vi "EnableDisable RTM.vi"(11 "Node Ptr":T1 format="%.0x") -> ()   [LabVIEW 2020, in "Ballard ARINC 429 System Explorer.lvlib" / "Implementation.lvlib"]
uses:
  Implementation.lvlib
  <vilib>/NI VeriStand/Custom Device API/Custom Device Item Ref.ctl
  Scripting/Ballard/Constants.vi
  <vilib>/NI VeriStand/Custom Device API/Custom Device API.lvlib
  Scripting/Ballard/Ballard ARINC 429 Scripting.lvlib
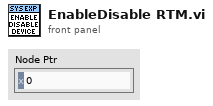
[diagram p1: front panel]
types:
  T1 = typedef "Custom Device API.lvlib/Custom Device Item Ref.ctl" = u64
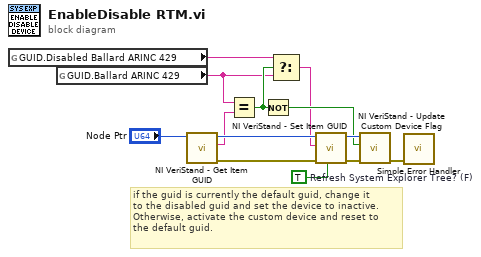
[diagram p0: block diagram]
diagram:
  w1 = TRUE  # Refresh System Explorer Tree? (F)
  # "if the guid is currently the default guid, change it \nto the disabled guid and set the device to inactive. \nOtherwise, activate the custom device and reset to \nthe default guid."
  n1 = global read "Constants.vi" "GUID.Disabled Ballard ARINC 429"() -> (w4:string)
  n2 = global read "Constants.vi" "GUID.Ballard ARINC 429"() -> (w3:string)
  n3 = call <vilib>:"NI VeriStand - Get Item GUID.vi"("Item Ref in"="Node Ptr") -> ("error out"=w9:errorcluster, "GUID"=w7:string, "Item Ref out"=w10:T1)  [unwired: 8 in]
  n4 = Equal?(x=w3, y=w7) -> (x = y?=w6:bool)
  n5 = Not(x=w6) -> (.not. x?=w5:bool)
  n6 = Select(t=w4, s=w6, f=w3) -> (s? t:f=w2:string)
  n7 = call <vilib>:"NI VeriStand - Set Item GUID.vi"("Refresh System Explorer Tree? (F)"=w1, "error in (no error)"=w9, "GUID"=w2, "Item Ref in"=w10) -> ("error out"=w8:errorcluster, "Item Ref out"=w11:T1)  [unwired: 6 in]
  n8 = call <vilib>:"NI VeriStand - Update Custom Device Flag.vi"("error in (no error)"=w8, "Is Custom Device Active?"=w5, "Device Ref in"=w11) -> ("error out"=w12:errorcluster)  [unwired: 7 in, 1 out]
  n9 = call <vilib>:"Simple Error Handler.vi"("error in (no error)"=w12) -> ()  [unwired: 4 in, 5 out]
